vi "Teleop.vi"(10 "Match Info":T1={"Autonomous Elapsed Seconds"=0.0, "TeleOp Elapsed Seconds"=0.0, "Disabled Elapsed Seconds"=0.0, "Visited Autonomous"=FALSE, "Visited TeleOp"=FALSE, "Visited Disabled"=FALSE, "Autonomous Settings"={"Autonomous Style"=enum."Independent", "VI Refnum"=refnum}}, 11 "Call Context":T2) -> ()   [LabVIEW 2014]
doc: "This VI is called for each TeleOp packet received from the DS where the robot is not disabled. It is often used to read from the joysticks and update I/O or to update setpoints for timed control loops. It should complete and return within 20 milliseconds or it may miss DS packets."
uses:
  <vilib>/Rock Robotics/WPI/DriverStation/WPI_DriverStationDerivedRobotMode.ctl
  <vilib>/Rock Robotics/WPI/DriverStation/WPI_DriverStationMatch Info.ctl
  <vilib>/Rock Robotics/WPI/Joystick/WPI_JoystickGetSetRefNum.vi
  <vilib>/Rock Robotics/Network Tables/SD Write Boolean Array.vi
  <vilib>/Rock Robotics/Network Tables/SD Write Numeric Array.vi
  <vilib>/Rock Robotics/Network Tables/SD Read Boolean.vi
  <vilib>/Rock Robotics/Network Tables/SD Read Number.vi
  <vilib>/Rock Robotics/WPI/RobotDrive/WPI_RobotDriveGetSetRefNum.vi
panel:
  out "Angle":u16
  out "Sample Slider 0":dbl(slide) scale=0.0..5.0
  out "Sample Boolean 1":bool
  out "Sample Boolean 0":bool
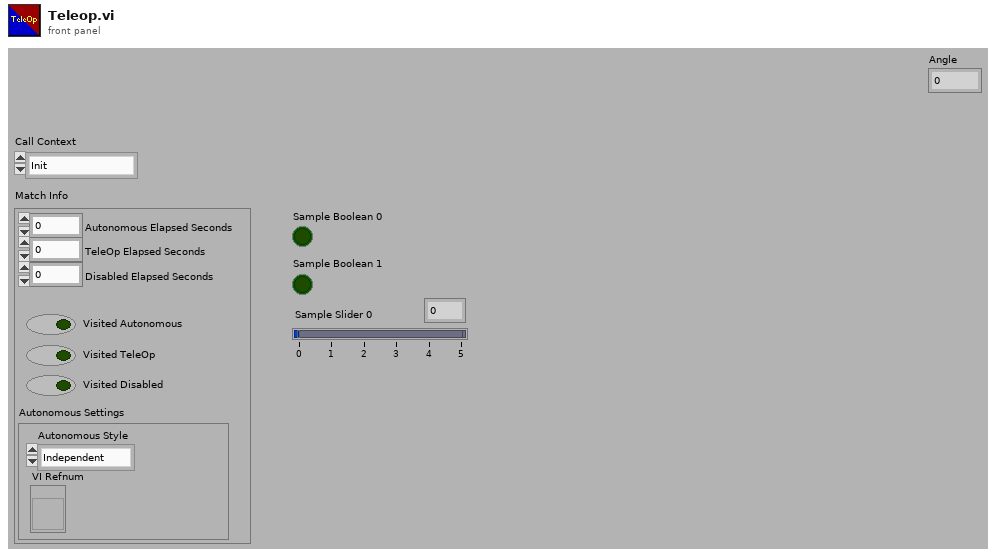
[diagram p1: front panel]
types:
  T1 = typedef "WPI_DriverStationMatch Info.ctl" = cluster{"Autonomous Elapsed Seconds":dbl, "TeleOp Elapsed Seconds":dbl, "Disabled Elapsed Seconds":dbl, "Visited Autonomous":bool, "Visited TeleOp":bool, "Visited Disabled":bool, "Autonomous Settings":cluster{"Autonomous Style":enum16{"Iterative", "Independent"}, "VI Refnum":refnum<vi>}}
  T2 = typedef "WPI_DriverStationDerivedRobotMode.ctl" = enum16{"Init", "Execute", "Stop"}
  T3 = typedef "WPI_JoystickDevRef.ctl" = cluster{"Device":T4}
  T4 = typedef "WPI_JoystickDeviceEnum.ctl" = enum16{"USB 0", "USB 1", "USB 2", "USB 3", "USB 4", "USB 5"}
  T5 = cluster{"Buttons[0]":bool, "Buttons[1]":bool, "Buttons[2]":bool, "Buttons[3]":bool, "Buttons[4]":bool, "Buttons[5]":bool, "Buttons[6]":bool, "Buttons[7]":bool, "Buttons[8]":bool}
  T6 = cluster{"Axes[0]":dbl, "Axes[1]":dbl, "Axes[2]":dbl, "Axes[3]":dbl, "Axes[4]":dbl, "Axes[5]":dbl, "Axes[6]":dbl, "Axes[7]":dbl, "Axes[8]":dbl}
  T7 = typedef "WPI_RobotDriveDevRef.ctl" = cluster{"DevStatus":errorcluster, "Motors[]":T8[], "Square Inputs":bool, "Max Output":dbl}
  T8 = typedef "WPI_MotorControlDeviceRef.ctl" = cluster{"DeviceStatus":errorcluster, "Type":T9, "PWM":cluster{"Controller":T10, "PWM Channel":T11, "DeadBand":T12}, "CAN":cluster{"Device Number":u8, "Control Mode":T13, "Semaphore":T14, "Max Vout":dbl, "TalonSRX Control Mode":T15}, "Invert":bool, "TransformRef":T16, "InvTransformRef":T16}
  T9 = typedef "WPI_MotorControlType.ctl" = enum16{"PWM", "CAN", "CANTalonSRX"}
  T10 = typedef "FPGA_TypedefDigitalModule.ctl" = enum16{"Controller 1"}
  T11 = typedef "FPGA_DIOPWMChannel.ctl" = enum8{"PWM 0", "PWM 1", "PWM 2", "PWM 3", "PWM 4", "PWM 5", "PWM 6", "PWM 7", "PWM 8", "PWM 9", "PWM MXP 0", "PWM MXP 1", "PWM MXP 2", "PWM MXP 3", "PWM MXP 4", "PWM MXP 5", "PWM MXP 6", "PWM MXP 7", "PWM MXP 8", "PWM MXP 9", "Invalid"}
  T12 = typedef "WPI_PWMDeadband.ctl" = cluster{"Name":string, "maxPositivePwm":i32, "minPositivePwm":i32, "centerPwm":i32, "maxNegativePwm":i32, "minNegativePwm":i32, "angularRange":u16}
  T13 = typedef "WPI_CANJaguar_ControlMode.ctl" = enum8{"Percent VBus", "Current", "Speed", "Position", "Voltage"}
  T14 = typedef "Semaphore RefNum" = refnum<k1>
  T15 = typedef "WPI_CANTalonSRX_APIControlMode.ctl" = enum8{"Percent VBus", "Speed", "Position", "Slave", "Unchanged / Invalid"}
  T16 = typedef "WPI_PWMTransform_ConPane.ctl" = refnum<vi>
  T17 = typedef "WPI_ServoDeviceRef.ctl" = cluster{"DeviceStatus":errorcluster, "Controller":T10, "PWM Channel":T11, "DeadBand":T12}
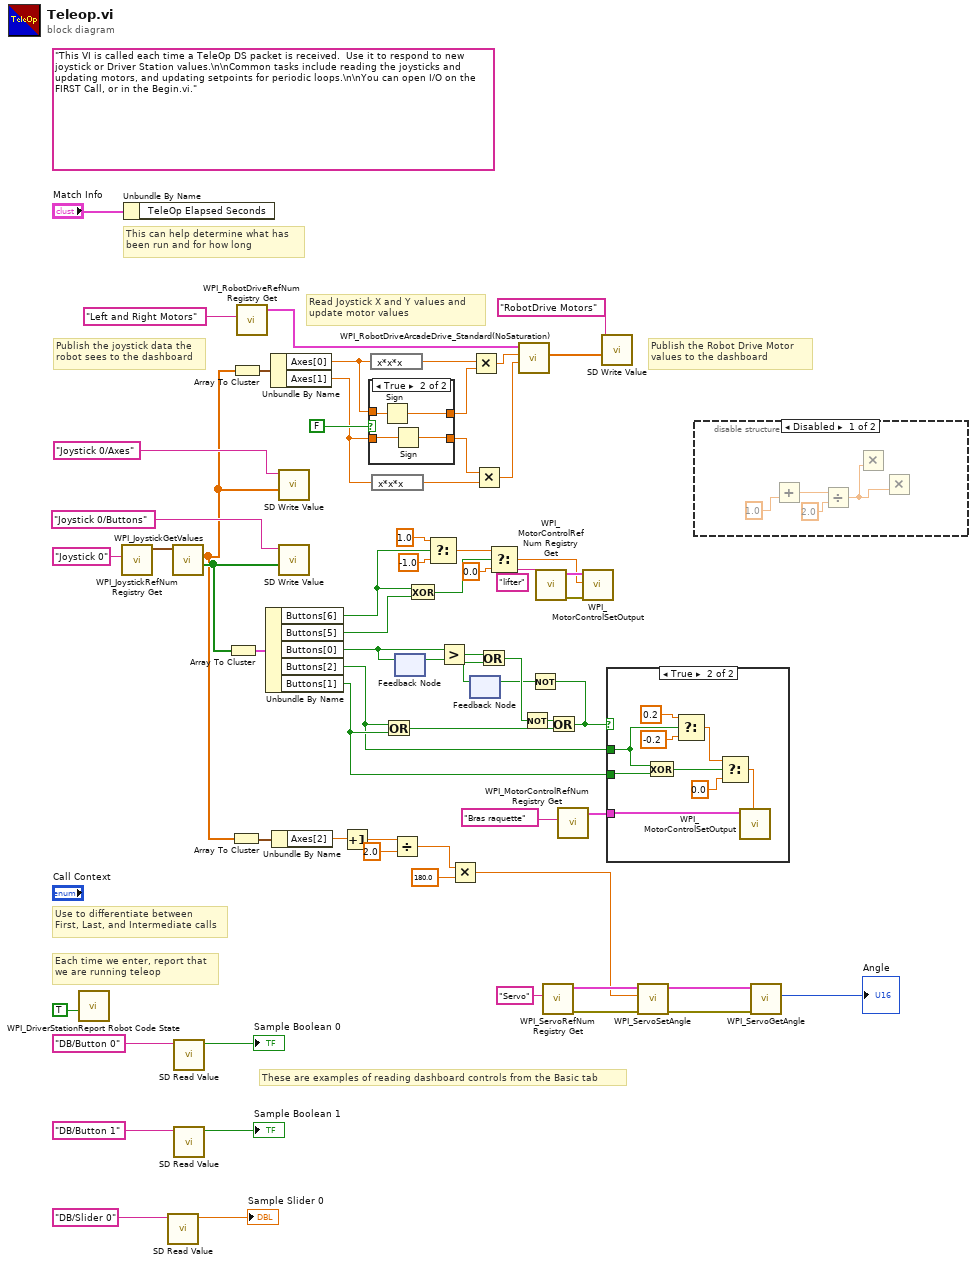
[diagram p0: block diagram]
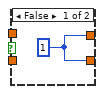
[diagram p2: hidden frame]
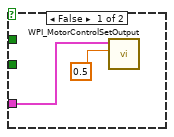
[diagram p3: hidden frame]
diagram:
  (unwired) "This VI is called each time a TeleOp DS packet is received.  Use it to respond to new joystick or Driver Station values.\n\nCommon tasks include reading the joysticks and updating motors, and updating setpoints for periodic loops.\n\nYou can open I/O on the FIRST Call, or in the Begin.vi."
  # "These are examples of reading dashboard controls from the Basic tab"
  # "Publish the Robot Drive Motor\nvalues to the dashboard"
  # "Publish the joystick data the\nrobot sees to the dashboard"
  # "Each time we enter, report that\nwe are running teleop"
  # "Use to differentiate between\nFirst, Last, and Intermediate calls"
  # "This can help determine what has\nbeen run and for how long"
  # "Read Joystick X and Y values and \nupdate motor values"
  n1 = call <vilib>:"WPI_DriverStationReport Robot Code State.vi"("TeleOp"=TRUE ("Autonomous")) -> ()  [unwired: 10 in, 1 out]
  n2 = call <vilib>:"WPI_JoystickRefNum Registry Get.vi"("refnum name"="Joystick 0") -> ("JoystickDevRef"=w62:T3)  [unwired: 1 in, 9 out]
  n3 = Unbundle By Name("Match Info") -> ()  [unwired: 1 out]
  n4 = call-poly <vilib>:"SD Read Value.vi"("Name"="DB/Slider 0" ("refnum name")) -> ("Numeric"=→"Sample Slider 0":dbl)  [unwired: 8 in, 2 out]
  n5 = call <vilib>:"WPI_JoystickGetValues.vi"("JoystickDevRef"=w62) -> ("Buttons"=w41:bool[], "Axes"=w13:dbl[])  [unwired: 6 in, 3 out]
  n6 = call-poly <vilib>:"SD Read Value.vi"("Name"="DB/Button 0" ("refnum name")) -> ("Boolean"=→"Sample Boolean 0":bool)  [unwired: 8 in, 2 out]
  n7 = call-poly <vilib>:"SD Read Value.vi"("Name"="DB/Button 1" ("refnum name")) -> ("Boolean"=→"Sample Boolean 1":bool)  [unwired: 8 in, 2 out]
  n8 = Array To Cluster(array=w41) -> (cluster=w40:T5)
  n9 = Array To Cluster(array=w13) -> (cluster=w12:T6)
  n10 = Array To Cluster(array=w13) -> (cluster=w19:T6)
  n11 = call <vilib>:"WPI_RobotDriveRefNum Registry Get.vi"("refnum name"="Left and Right Motors") -> ("RobotDriveDevRef"=w64:T7)  [unwired: 1 in, 9 out]
  n12 = Unbundle By Name(w40) -> ("Buttons[6]"=w38:bool, "Buttons[5]"=w39:bool, "Buttons[0]"=w28:bool, "Buttons[2]"=w29:bool, "Buttons[1]"=w30:bool)
  n13 = Unbundle By Name(w19) -> ("Axes[0]"=w18:dbl, "Axes[1]"=w16:dbl)
  n14 = Unbundle By Name(w12) -> ("Axes[2]"=w11:dbl)
  n15 = call-poly <vilib>:"SD Write Value.vi"("Numeric Array"=w13, "Name"="Joystick 0/Axes") -> ()  [unwired: 8 in, 2 out]
  n16 = call-poly <vilib>:"SD Write Value.vi"("Boolean Array"=w41, "Name"="Joystick 0/Buttons") -> ()  [unwired: 8 in, 2 out]
  n17 = Increment(x=w11) -> (x+1=w9:dbl)
  n18 = case shown="True" FALSE {
    tunnel: [w67 w71] -> w35
    tunnel: w16 -> [_ w70]
    tunnel: w18 -> [_ w69]
    tunnel: [w67 w68] -> w15
    frame False {
      w67 = 1
    }
    frame True {
      n19 = Sign(1:w69) -> (0:w71:dbl)
      n20 = Sign(1:w70) -> (0:w68:dbl)
    }
  }
  n21 = expression code="x*x*x"(w18) -> (w37:dbl)
  n22 = expression code="x*x*x"(w16) -> (w36:dbl)
  n23 = Or(x=w29, y=w30) -> (x .or. y?=w22:bool)
  n24 = Divide(x=w9, y=2.0) -> (x/y=w7:dbl)
  n25 = feedback-in #1(w28) -> ()
  n26 = feedback #1() -> (w27:bool)  [unwired: 1 in]
  n27 = Exclusive Or(1:w39, 2:w38) -> (0:w44:bool)
  n28 = Select(t=1.0, s=w38, f=-1.0) -> (s? t:f=w43:dbl)
  n29 = Greater?(x=w28, y=w27) -> (0:w26:bool)
  n30 = Multiply(x=w7, y=180.0) -> (x*y=w5:dbl)
  n31 = feedback #2() -> (w23:bool)  [unwired: 1 in]
  n32 = Multiply(x=w37, y=w35) -> (x*y=w34:dbl)
  n33 = Multiply(x=w15, y=w36) -> (x*y=w33:dbl)
  n34 = Or(x=w26, y=w23) -> (x .or. y?=w24:bool)
  n35 = Select(t=w43, s=w44, f=0.0) -> (s? t:f=w42:dbl)
  n36 = call <vilib>:"WPI_RobotDriveArcadeDrive_Standard(NoSaturation).vi"("Y axis value"=w33, "X axis value"=w34, "RobotDriveDevRef"=w64) -> ("Motor Values"=w53:dbl[])  [unwired: 1 in, 7 out]
  n37 = Not(x=w24) -> (.not. x?=w25:bool)
  n38 = call <vilib>:"WPI_MotorControlRefNum Registry Get.vi"("refnum name"="lifter") -> ("error out"=w48:errorcluster, "MotorControlDevRef"=w49:T8)  [unwired: 9 in]
  n39 = call <vilib>:"WPI_ServoRefNum Registry Get.vi"("refnum name"="Servo") -> ("error out"=w2:errorcluster, "ServoDeviceRef"=w10:T17)  [unwired: 9 in]
  n40 = Or(x=w25, y=w22) -> (x .or. y?=w21:bool)
  n41 = Not(x=w21) -> (.not. x?=w20:bool)
  n42 = feedback-in #2(w20) -> ()
  n43 = call <vilib>:"WPI_MotorControlRefNum Registry Get.vi"("refnum name"="Bras raquette") -> ("MotorControlDevRef"=w32:T8)  [unwired: 9 in, 1 out]
  n44 = call <vilib>:"WPI_MotorControlSetOutput.vi"("error in (no error)"=w48, "Output"=w42, "MotorControlDevRef"=w49) -> ()  [unwired: 6 in, 3 out]
  n45 = call-poly <vilib>:"SD Write Value.vi"("Numeric Array"=w53, "Name"="RobotDrive Motors") -> ()  [unwired: 8 in, 2 out]
  n46 = case shown="True" w21 {
    tunnel: w32 -> [w73 w77]
    tunnel: w29 -> [_ w74]
    tunnel: w30 -> [_ w75]
    frame False {
      n47 = call <vilib>:"WPI_MotorControlSetOutput.vi"("Output"=0.5, "MotorControlDevRef"=w73) -> ()  [unwired: 7 in, 3 out]
    }
    frame True {
      n48 = Exclusive Or(1:w75, 2:w74) -> (0:w79:bool)
      n49 = Select(t=0.2, s=w74, f=-0.2) -> (s? t:f=w78:dbl)
      n50 = Select(t=w78, s=w79, f=0.0) -> (s? t:f=w76:dbl)
      n51 = call <vilib>:"WPI_MotorControlSetOutput.vi"("Output"=w76, "MotorControlDevRef"=w77) -> ()  [unwired: 7 in, 3 out]
    }
  }
  n52 = call <vilib>:"WPI_ServoSetAngle.vi"("error in (no error)"=w2, "Angle"=w5, "ServoDeviceRef"=w10) -> ("error out"=w1:errorcluster, "ServoDeviceRef"=w4:T17)  [unwired: 7 in]
  n53 = disable-structure shown="Disabled" {
    frame Disabled {
      n54 = Add(y=1.0) -> (x=w85:dbl, x+y=w88:dbl)
      n55 = Divide(x=w88, y=2.0 ("x/y")) -> (x/y=w84:dbl)
      n56 = Multiply(y=w84) -> (x=w83:dbl)  [unwired: 1 out]
      n57 = Multiply(y=w84) -> (x=w89:dbl)  [unwired: 1 out]
    }
    frame Enabled {
    }
  }
  n58 = call <vilib>:"WPI_ServoGetAngle.vi"("ServoDeviceRef"=w4, "error in (no error)"=w1) -> ("Angle"=→"Angle":u16)  [unwired: 6 in, 2 out]
